vi "Create Client.vi"(8 "error in":errorcluster, 10 "certificatePath":string, 11 "address":string) -> (0 "error out":errorcluster, 3 "gRPC ID Out":T1)   [LabVIEW 2019, in "Example_2_client.lvlib"]
uses:
  Example_2_client.lvlib
  <vilib>/gRPC/LabVIEW gRPC Library/grpc-lvsupport-release.lvlib
  <vilib>/gRPC/LabVIEW gRPC Library/Shared/grpcId.ctl
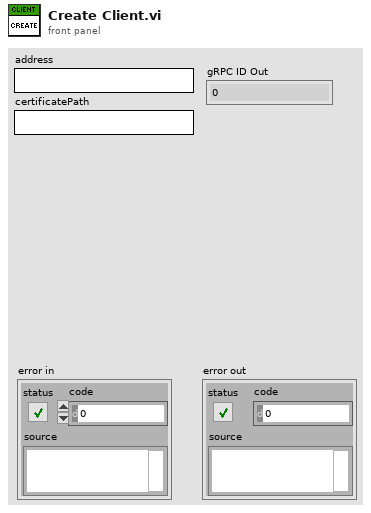
[diagram p1: front panel]
types:
  T1 = typedef "grpc-lvsupport-release.lvlib/grpcId.ctl" = u64
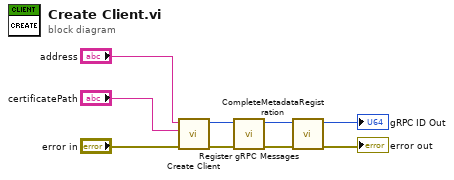
[diagram p0: block diagram]
diagram:
  n1 = call <vilib>:"Create Client.vi"("error in"="error in", "certificatePath"="certificatePath", "address"="address") -> ("error out"=w5:errorcluster, "ClientID out"=w4:T1)  [unwired: 7 in]
  n2 = call "Register gRPC Messages.vi"("error in (no error)"=w5, "gRPC ID"=w4) -> ("error out"=w2:errorcluster, "gRPC ID Out"=w3:T1)  [unwired: 8 in]
  n3 = call <vilib>:"CompleteMetadataRegistration.vi"("error in"=w2, "gRPC ID in"=w3) -> ("error out"=→"error out":errorcluster, "gRPC ID Out"=→"gRPC ID Out":T1)  [unwired: 8 in]
